vi "Terminate.vi"(8 "error in (no error)":errorcluster, 10 "Message in":refnum<class "TerminateMessage.lvclass">, 11 "Galvo in":refnum<class "ImagingModeSPIM.lvclass">) -> (0 "error out":errorcluster, 3 "Galvo out":refnum<class "ImagingModeSPIM.lvclass">)   [LabVIEW 2012, in "ImagingModeSPIM.lvclass"]
doc: "This member function is called when the statemachine in the run.vi receives an 'terminate' command. It closes the RabbitMQ connection. \n\nOverride this member function in your derived class to release all previously acquired resources (but don't forget to call the parent method). If your component has subcomponents, they count as resources, and you have to release them by calling their own terminate functions."
uses:
  ImagingModeSPIM.lvclass
  <vilib>/Distrio/Murmex/TerminateMessage/TerminateMessage.lvclass
  ImagingModeSPIM.lvclass/ImagingModeSPIM.ctl
  <vilib>/Distrio/Murmex/Murmex/Murmex.lvclass
panel:
  # "This method is called when the TERMINATE\ntrigger is sent. \n\nOverride this method when your component needs to\nrespond to this trigger. \n\nCall parent for proper implementation"
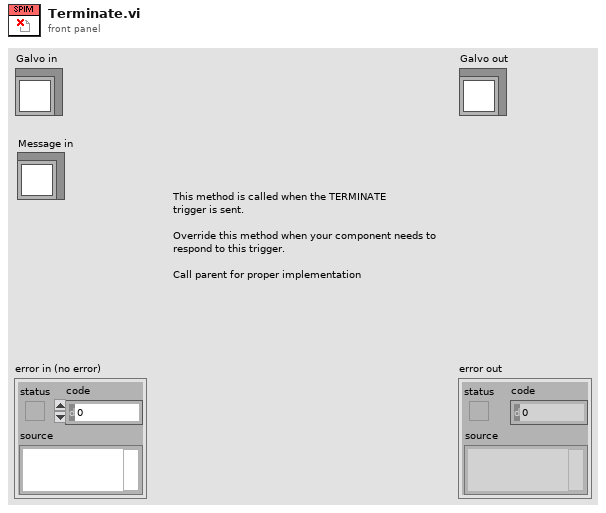
[diagram p1: front panel]
types:
  T1 = enum8{"Enabled", "Disabled", "Disabled and Grayed Out"}
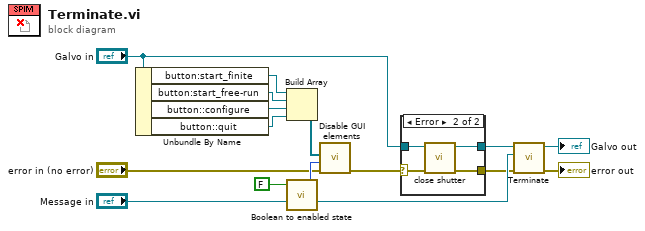
[diagram p0: block diagram]
diagram:
  n1 = Unbundle By Name("Galvo in") -> ("button:start_finite"=w6:refnum<vi>, "button:start_free-run"=w7:refnum<vi>, "button::configure"=w8:refnum<vi>, "button::quit"=w9:refnum<vi>)
  n2 = Build Array(w6, w7, w8, w9) -> (w5:refnum<vi>[])
  n3 = call <vilib>:"Boolean to enabled state.vi"("boolean in"=FALSE) -> ("enabled status out"=w11:T1)  [unwired: 4 in]
  n4 = call <vilib>:"Disable GUI elements.vi"("error in (no error)"="error in (no error)", "enabled state"=w11, "control refs"=w5) -> ("error out"=w4:errorcluster)  [unwired: 8 in]
  n5 = case shown="Error" w4 {
    selector: w4 -> [w17 w21]
    tunnel: [w17 w20] -> w3
    tunnel: "Galvo in" -> [w16 w19]
    tunnel: [w16 w18] -> w1
    frame No Error {
    }
    frame Error {
      n6 = call "close shutter.vi"("error in (no error)"=w21, "Murmex in"=w19) -> ("error out"=w20:errorcluster, "Murmex out"=w18:refnum<class "ImagingModeSPIM.lvclass">)  [unwired: 8 in]
    }
  }
  n7 = call-parent "Terminate.vi"("error in (no error)"=w3, "Message in"="Message in", "Murmex in"=w1) -> ("error out"=→"error out":errorcluster, "Murmex out"=→"Galvo out":refnum<class "ImagingModeSPIM.lvclass">)  [unwired: 7 in]
